vi "Test Write.vi"(8 "error in (no error)":errorcluster, 11 "RemoteControl.ZMQ in":refnum<class "RemoteControl.ZMQ.lvclass">) -> (0 "error out":errorcluster, 3 "RemoteControl.ZMQ out":refnum<class "RemoteControl.ZMQ.lvclass">)   [LabVIEW 2019, in "RemoteControl.ZMQ.lvclass"]
uses:
  RemoteControl.ZMQ.lvclass
  <vilib>/addons/zeromq/zmq_socket.lvclass
  <vilib>/addons/zeromq/socket_type.ctl
  <vilib>/addons/_JKI Toolkits/Caraya/classes/Assert/Assert Not Error.vi
  <vilib>/addons/_JKI Toolkits/Caraya/classes/Assert/Assert Error.vi
  <vilib>/addons/_JKI Toolkits/Caraya/classes/Assert/Assert.lvclass
  <vilib>/addons/zeromq/zmq_context.lvclass
  <vilib>/addons/zeromq/zeromq.lvlib
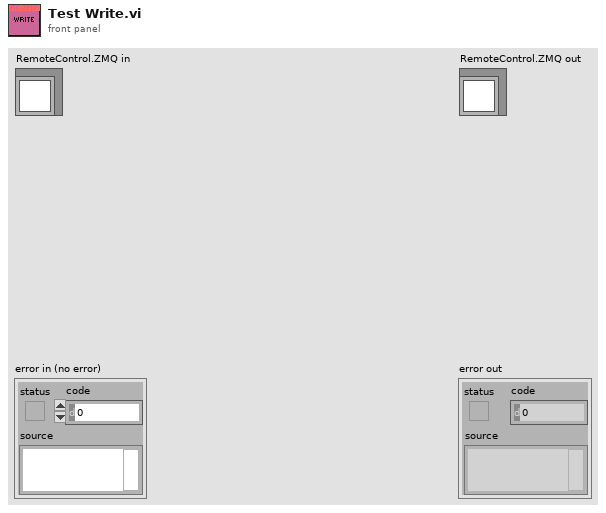
[diagram p1: front panel]
types:
  T1 = typedef "zeromq.lvlib/socket_type.ctl" = enum8{"ZMQ_PAIR", "ZMQ_PUB", "ZMQ_SUB", "ZMQ_REQ", "ZMQ_REP", "ZMQ_DEALER", "ZMQ_ROUTER", "ZMQ_PULL", "ZMQ_PUSH", "ZMQ_XPUB", "ZMQ_XSUB", "ZMQ_STREAM", "ZMQ_SERVER", "ZMQ_CLIENT", "ZMQ_RADIO", "ZMQ_DISH", "ZMQ_GATHER", "ZMQ_SCATTER", "ZMQ_DGRAM"}
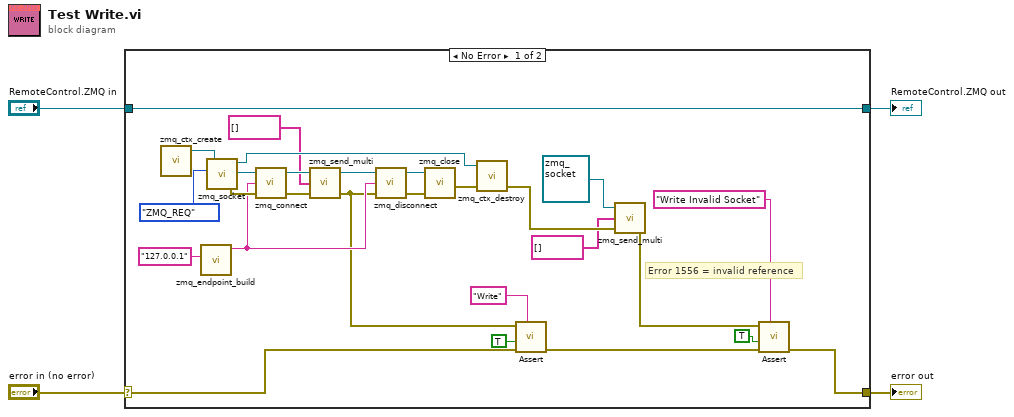
[diagram p0: block diagram]
diagram:
  n1 = case shown="No Error" "error in (no error)" {
    selector: "error in (no error)" -> [w16 w33]
    tunnel: [w31 w33] -> w3
    tunnel: [w28 w32] -> w1
    tunnel: "RemoteControl.ZMQ in" -> [w28 w32]
    frame No Error {
      # "Error 1556 = invalid reference"
      n2 = call <vilib>:"zmq_ctx_create.vi"() -> ("context out"=w25:refnum<class "zmq_context.lvclass">)  [unwired: 4 in, 1 out]
      n3 = call <vilib>:"zmq_endpoint_build.vi"("address"="127.0.0.1") -> ("endpoint"=w11:string)  [unwired: 4 in, 2 out]
      n4 = call <vilib>:"zmq_socket.vi"("socket type"=socket_type."ZMQ_REQ", "context in"=w25) -> ("error out"=w24:errorcluster, "socket out"=w23:refnum<class "zmq_socket.lvclass">, "context out"=w18:refnum<class "zmq_context.lvclass">)  [unwired: 3 in]
      n5 = call <vilib>:"zmq_connect.vi"("error in"=w24, "endpoint"=w11, "socket in"=w23) -> ("error out"=w10:errorcluster, "socket out"=w9:refnum<class "zmq_socket.lvclass">)  [unwired: 1 in]
      n6 = call <vilib>:"zmq_send_multi.vi"("error in"=w10, "parts"=string[] [], "socket in"=w9) -> ("error out"=w6:errorcluster, "socket out"=w7:refnum<class "zmq_socket.lvclass">)  [unwired: 1 in]
      n7 = call <vilib>:"zmq_disconnect.vi"("error in"=w6, "endpoint"=w11, "socket in"=w7) -> ("error out"=w21:errorcluster, "socket out"=w20:refnum<class "zmq_socket.lvclass">)  [unwired: 1 in]
      n8 = call <vilib>:"zmq_close.vi"("error in"=w21, "socket"=w20) -> ("error out"=w19:errorcluster)  [unwired: 3 in]
      n9 = call <vilib>:"zmq_ctx_destroy.vi"("error in"=w19, "context in"=w18) -> ("error out"=w15:errorcluster)  [unwired: 3 in]
      n10 = call-poly <vilib>:"Assert.vi"("Label"="Write", "error in (no error)"=w16, "Register with caller test (F)"=TRUE, "Not Error?"=w6) -> ("error out"=w14:errorcluster)  [unwired: 7 in]
      n11 = call <vilib>:"zmq_send_multi.vi"("error in"=w15, "parts"=string[] [], "socket in"=refnum<class "zmq_socket.lvclass"> refnum) -> ("error out"=w26:errorcluster)  [unwired: 1 in, 1 out]
      n12 = call-poly <vilib>:"Assert.vi"("Label"="Write Invalid Socket", "error in (no error)"=w14, "Register with caller test (F)"=TRUE, "Error?"=w26) -> ("error out"=w31:errorcluster)  [unwired: 7 in]
    }
    frame Error {
    }
  }
  "error out" <- w3
  "RemoteControl.ZMQ out" <- w1
